vi "Boceto programa final.vi"() -> ()   [LabVIEW 2014]
panel:
  out "Gráfica":waveform(dbl)(graph)
  in  "Canal MATH":bool
  in  "VISA resource name":refnum<visa-resource-name>
  in  "Canal 1":bool
  in  "Canal 2":bool
  out "error out":errorcluster
  out "VISA resource name out":refnum<visa-resource-name>
  in  "error in (no error)":errorcluster
  out "Comando 4":string
  out "Medidas":string
  out "Comando 2":string
  out "Comando 1":string
  in  "Estilo de onda":u16(ring) items=["Puntos", "Vectores"]
  in  "Invertir colores":bool
  in  "Formato (YT o XY)":u16(ring) items=["YT", "XY"]
  in  "Contraste":i32(knob)=63 scale=0.0..100.0
  in  "Invertir canal":bool
  in  "Posición horizontal":i32(knob) scale=-5.0..5.0
  in  "Posición vertical":i32(knob) scale=-5.0..5.0
  in  "Escala vertical (V)":u16(ring) items=["2 mV", "5 mV", "10 mV", "20 mV", "50  mV", "100 mV", "200 mV", "500 mV", "1 V", "2 V", "5 V"]
  in  "Escala horizontal (s)":u16(ring) items=["25 n", "50 n", "100 n", "250 n", "500 n", "1 u", "2,5 u", "5 u", "10 u", "25 u", "50 u", "100 u", "250 u", "500 u", "1 m", "2,5 m", "5 m", "10 m", "25 m", "50 m", "100 m", "250 m", "500 m", "1 ", "2,5", "5", "10", "25", "50"]
  in  "Operaciones \ncon las señales":u16(ring)=1 items=["CH1 + CH2"=1, "CH1 - CH2"=2, "CH2 - CH1"=3, "CH1 * CH2"=4]
  in  "Acomplamiento":u16(ring) items=["AC", "DC", "GROUND"]
  in  "Selección de canal":u16(ring) items=["Canal 1", "Canal 2"]
  in  "Atenuación":u16(ring) items=["x1", "x10", "x20", "x50", "x100", "x500", "x1000"]
  in  "Ancho de banda":u16(ring)=1 items=["ON", "OFF"]
  out "Selección canal":string
  out "Comando concatenado":string
  in  "stop":bool
  out "Comando final":string
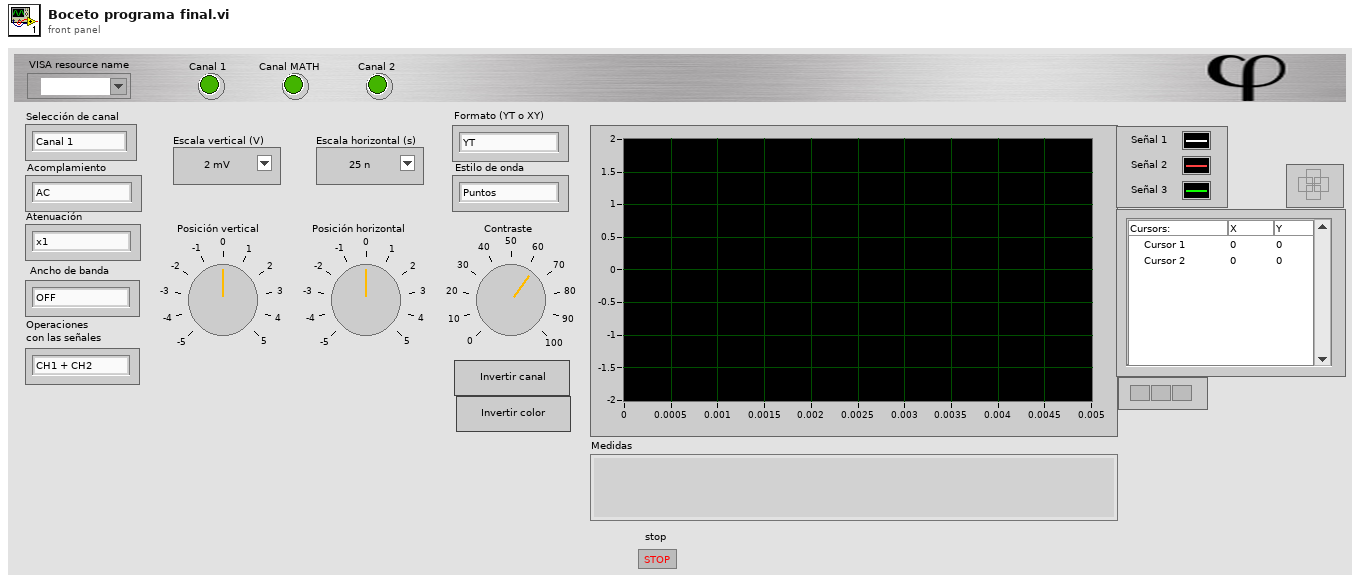
[diagram p1: front panel]
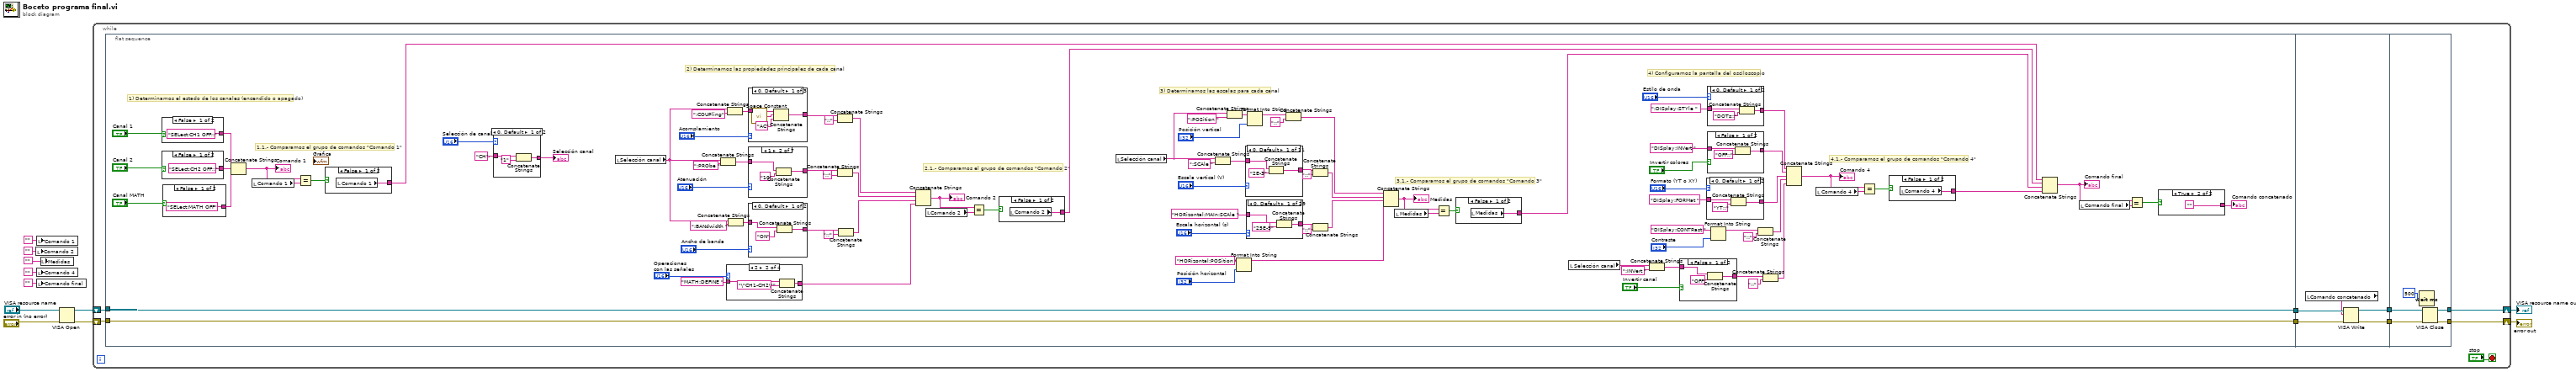
[diagram p0: block diagram]
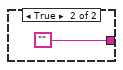
[diagram p2: hidden frame]
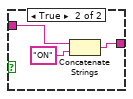
[diagram p3: hidden frame]
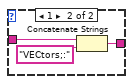
[diagram p4: hidden frame]
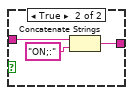
[diagram p5: hidden frame]
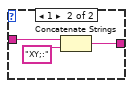
[diagram p6: hidden frame]
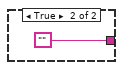
[diagram p7: hidden frame]
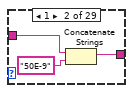
[diagram p8: hidden frame]
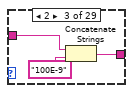
[diagram p9: hidden frame]
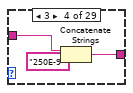
[diagram p10: hidden frame]
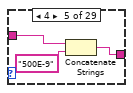
[diagram p11: hidden frame]
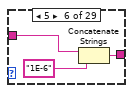
[diagram p12: hidden frame]
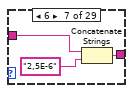
[diagram p13: hidden frame]
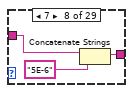
[diagram p14: hidden frame]
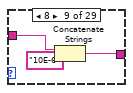
[diagram p15: hidden frame]
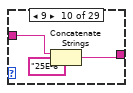
[diagram p16: hidden frame]
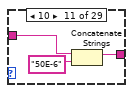
[diagram p17: hidden frame]
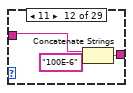
[diagram p18: hidden frame]
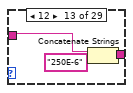
[diagram p19: hidden frame]
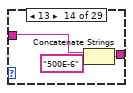
[diagram p20: hidden frame]
diagram:
  n1 = local write "Comando 2"("") -> ()
  n2 = local write "Comando 1"("") -> ()
  n3 = local write "Comando 4"("") -> ()
  n4 = local write "Comando final"("") -> ()
  n5 = local write "Medidas"("") -> ()
  n6 = VISA Open(error in (no error)="error in (no error)", VISA resource name="VISA resource name") -> (VISA resource name=w11:refnum<visa-resource-name>, error out=w10:errorcluster)  [unwired: 3 in]
  n7 = while {
    shift-right: [w13] -> w9
    shift-left: w11 -> [w18]
    shift-right: [w12] -> w8
    shift-left: w10 -> [w17]
    stop <- "stop" stop-if-true
    n8 = flat-sequence {
      tunnel: w18 -> [w114]
      tunnel: w17 -> [w113]
      tunnel: [w114] -> w20
      tunnel: [w113] -> w19
      tunnel: [w333] -> w15
      tunnel: w19 -> [w336]
      tunnel: w20 -> [w337]
      tunnel: [w334] -> w14
      tunnel: w15 -> [w338]
      tunnel: w14 -> [w339]
      tunnel: [w339] -> w13
      tunnel: [w338] -> w12
      frame #0 {
        # "1) Determinamos el estado de los canales (encendido o apagado)"
        # "4.1.- Comparamos el grupo de comandos \"Comando 4\""
        # "4) Configuramos la pantalla del osciloscopio"
        # "3.1.- Comparamos el grupo de comandos \"Comando 3\""
        # "3) Determinamos las escalas para cada canal"
        # "2.1.- Comparamos el grupo de comandos \"Comando 2\""
        # "1.1.- Comparamos el grupo de comandos \"Comando 1\""
        # "2) Determinamos las propiedades principales de cada canal"
        n9 = case shown="False" "Canal 1" {
          tunnel: ["SELect:CH1 OFF;:" "SELect:CH1 ON;:"] -> w107
          frame False {
          }
          frame True {
          }
        }
        n10 = case shown="False" "Canal 2" {
          tunnel: ["SELect:CH2 OFF;:" "SELect:CH2 ON;:"] -> w106
          frame False {
          }
          frame True {
          }
        }
        n11 = case shown="False" "Canal MATH" {
          tunnel: ["SELect:MATH OFF" "SELect:MATH ON"] -> w105
          frame False {
          }
          frame True {
          }
        }
        n12 = Concatenate Strings(w107, w106, w105) -> (w104:string)
        "Comando 1" <- w104
        n13 = local read "Comando 1"() -> (w103:string)
        n14 = Equal?(x=w104, y=w103) -> (x = y?=w102:bool)
        n15 = case shown="False" w102 {
          tunnel: [w317 ""] -> w33
          frame False {
            n16 = local read "Comando 1"() -> (w317:string)
          }
          frame True {
          }
        }
        n17 = case shown="0, Default" "Selección de canal" {
          tunnel: "CH" -> [w327 w330]
          tunnel: [w325 w328] -> w109
          frame 0, Default {
            n18 = Concatenate Strings(w327, "1") -> (w325:string)
          }
          frame 1 {
            n19 = Concatenate Strings(w330, "2") -> (w328:string)
          }
        }
        "Selección canal" <- w109
        n20 = local read "Selección canal"() -> (w84:string)
        n21 = Concatenate Strings(w84, ":PRObe ") -> (w98:string)
        n22 = case shown="2" "Operaciones \ncon las señales" {
          tunnel: "MATH:DEFINE " -> [w268 w271 w273 w276]
          tunnel: [w266 w270 w272 w275] -> w29
          frame 1, Default {
            n23 = Concatenate Strings(w268, "\"CH1+CH2\"") -> (w266:string)
          }
          frame 2 {
            n24 = Concatenate Strings(w271, "\"CH1-CH2\"") -> (w270:string)
          }
          frame 3 {
            n25 = Concatenate Strings(w273, "\"CH2-CH1\"") -> (w272:string)
          }
          frame 4 {
            n26 = Concatenate Strings(w276, "\"CH1*CH2\"") -> (w275:string)
          }
        }
        n27 = Concatenate Strings(w84, ":COUPling") -> (w101:string)
        n28 = Concatenate Strings(w84, ":BANdwidth ") -> (w96:string)
        n29 = case shown="1" "Atenuación" {
          tunnel: w98 -> [w285 w289 w291 w294 w297 w300 w303]
          tunnel: [w284 w287 w290 w293 w296 w299 w302] -> w87
          frame 0, Default {
            n30 = Concatenate Strings(w285, "1") -> (w284:string)
          }
          frame 1 {
            n31 = Concatenate Strings(w289, "10") -> (w287:string)
          }
          frame 2 {
            n32 = Concatenate Strings(w291, "20") -> (w290:string)
          }
          frame 3 {
            n33 = Concatenate Strings(w294, "50") -> (w293:string)
          }
          frame 4 {
            n34 = Concatenate Strings(w297, "100") -> (w296:string)
          }
          frame 5 {
            n35 = Concatenate Strings(w300, "500") -> (w299:string)
          }
          frame 6 {
            n36 = Concatenate Strings(w303, "1000") -> (w302:string)
          }
        }
        n37 = case shown="0, Default" "Ancho de banda" {
          tunnel: w96 -> [w280 w283]
          tunnel: [w278 w281] -> w85
          frame 0, Default {
            n38 = Concatenate Strings(w280, "ON") -> (w278:string)
          }
          frame 1 {
            n39 = Concatenate Strings(w283, "OFF") -> (w281:string)
          }
        }
        n40 = case shown="0, Default" "Acomplamiento" {
          tunnel: w101 -> [w306 w309 w314]
          tunnel: [w305 w310 w313] -> w90
          frame 0, Default {
            n41 = call <vilib>:"Space Constant.vi"() -> ("String"=w307:string)
            n42 = Concatenate Strings(w306, w307, "AC") -> (w305:string)
          }
          frame 1 {
            n43 = call <vilib>:"Space Constant.vi"() -> ("String"=w311:string)
            n44 = Concatenate Strings(w309, w311, "DC") -> (w310:string)
          }
          frame 2 {
            n45 = call <vilib>:"Space Constant.vi"() -> ("String"=w315:string)
            n46 = Concatenate Strings(w314, w315, "GND") -> (w313:string)
          }
        }
        n47 = Concatenate Strings(w90, ";:") -> (w28:string)
        n48 = Concatenate Strings(w87, ";:") -> (w27:string)
        n49 = Concatenate Strings(w85, ";:") -> (w26:string)
        n50 = Concatenate Strings(w28, w27, w26, w29) -> (w81:string)
        "Comando 2" <- w81
        n51 = local read "Comando 2"() -> (w82:string)
        n52 = Equal?(x=w81, y=w82) -> (x = y?=w83:bool)
        n53 = case shown="False" w83 {
          tunnel: [w264 ""] -> w32
          frame False {
            n54 = local read "Comando 2"() -> (w264:string)
          }
          frame True {
          }
        }
        n55 = local read "Selección canal"() -> (w67:string)
        n56 = Concatenate Strings(w67, ":SCAle ") -> (w71:string)
        n57 = Concatenate Strings(w67, ":POSition ") -> (w68:string)
        n58 = Format Into String(initial string="HORizontal:POSition ", "Posición horizontal") -> (resulting string=w76:string)  [unwired: 2 in, 1 out]
        n59 = case shown="0, Default" "Escala vertical (V)" {
          tunnel: w71 -> [w232 w236 w238 w241 w244 w247 w249 w253 w256 w259 w262]
          tunnel: [w231 w234 w237 w240 w243 w246 w250 w252 w255 w258 w261] -> w63
          frame 0, Default {
            n60 = Concatenate Strings(w232, "2E-3") -> (w231:string)
          }
          frame 1 {
            n61 = Concatenate Strings(w236, "5E-3") -> (w234:string)
          }
          frame 2 {
            n62 = Concatenate Strings(w238, "10E-3 ") -> (w237:string)
          }
          frame 3 {
            n63 = Concatenate Strings(w241, "20E-3") -> (w240:string)
          }
          frame 4 {
            n64 = Concatenate Strings(w244, "50E-3") -> (w243:string)
          }
          frame 5 {
            n65 = Concatenate Strings(w247, "100E-3") -> (w246:string)
          }
          frame 6 {
            n66 = Concatenate Strings(w249, "200E-3") -> (w250:string)
          }
          frame 7 {
            n67 = Concatenate Strings(w253, "500E-3") -> (w252:string)
          }
          frame 8 {
            n68 = Concatenate Strings(w256, "1") -> (w255:string)
          }
          frame 9 {
            n69 = Concatenate Strings(w259, "2") -> (w258:string)
          }
          frame 10 {
            n70 = Concatenate Strings(w262, "5") -> (w261:string)
          }
        }
        n71 = case shown="0, Default" "Escala horizontal (s)" {
          tunnel: "HORizontal:MAIn:SCAle " -> [w145 w149 w151 w154 w157 w160 w163 w166 w169 w172 w175 w177 w180 w183 w186 w189 w192 w195 w198 w201 w204 w207 w210 w213 w216 w219 w222 w225 w228]
          tunnel: [w144 w147 w150 w153 w156 w159 w164 w165 w168 w171 w174 w178 w181 w184 w187 w190 w193 w196 w199 w202 w205 w208 w211 w214 w217 w220 w223 w226 w229] -> w65
          frame 0, Default {
            n72 = Concatenate Strings(w145, "25E-9") -> (w144:string)
          }
          frame 1 {
            n73 = Concatenate Strings(w149, "50E-9") -> (w147:string)
          }
          frame 2 {
            n74 = Concatenate Strings(w151, "100E-9") -> (w150:string)
          }
          frame 3 {
            n75 = Concatenate Strings(w154, "250E-9") -> (w153:string)
          }
          frame 4 {
            n76 = Concatenate Strings(w157, "500E-9") -> (w156:string)
          }
          frame 5 {
            n77 = Concatenate Strings(w160, "1E-6") -> (w159:string)
          }
          frame 6 {
            n78 = Concatenate Strings(w163, "2,5E-6") -> (w164:string)
          }
          frame 7 {
            n79 = Concatenate Strings(w166, "5E-6") -> (w165:string)
          }
          frame 8 {
            n80 = Concatenate Strings(w169, "10E-6") -> (w168:string)
          }
          frame 9 {
            n81 = Concatenate Strings(w172, "25E-6") -> (w171:string)
          }
          frame 10 {
            n82 = Concatenate Strings(w175, "50E-6") -> (w174:string)
          }
          frame 11 {
            n83 = Concatenate Strings(w177, "100E-6") -> (w178:string)
          }
          frame 12 {
            n84 = Concatenate Strings(w180, "250E-6") -> (w181:string)
          }
          frame 13 {
            n85 = Concatenate Strings(w183, "500E-6") -> (w184:string)
          }
          frame 14 {
            n86 = Concatenate Strings(w186, "1E-3") -> (w187:string)
          }
          frame 15 {
            n87 = Concatenate Strings(w189, "2,5E-3") -> (w190:string)
          }
          frame 16 {
            n88 = Concatenate Strings(w192, "5E-3") -> (w193:string)
          }
          frame 17 {
            n89 = Concatenate Strings(w195, "10E-3") -> (w196:string)
          }
          frame 18 {
            n90 = Concatenate Strings(w198, "25E-3") -> (w199:string)
          }
          frame 19 {
            n91 = Concatenate Strings(w201, "50E-3") -> (w202:string)
          }
          frame 20 {
            n92 = Concatenate Strings(w204, "100E-3") -> (w205:string)
          }
          frame 21 {
            n93 = Concatenate Strings(w207, "250E-3") -> (w208:string)
          }
          frame 22 {
            n94 = Concatenate Strings(w210, "500E-3") -> (w211:string)
          }
          frame 23 {
            n95 = Concatenate Strings(w213, "1E0") -> (w214:string)
          }
          frame 24 {
            n96 = Concatenate Strings(w216, "2,5E0") -> (w217:string)
          }
          frame 25 {
            n97 = Concatenate Strings(w219, "5E0") -> (w220:string)
          }
          frame 26 {
            n98 = Concatenate Strings(w222, "10E0") -> (w223:string)
          }
          frame 27 {
            n99 = Concatenate Strings(w225, "25E0") -> (w226:string)
          }
          frame 28 {
            n100 = Concatenate Strings(w228, "50E0") -> (w229:string)
          }
        }
        n101 = Format Into String(initial string=w68, "Posición vertical") -> (resulting string=w74:string)  [unwired: 2 in, 1 out]
        n102 = Concatenate Strings(w74, ";:") -> (w24:string)
        n103 = Concatenate Strings(w63, ";:") -> (w25:string)
        n104 = Concatenate Strings(w65, ";:") -> (w64:string)
        n105 = Concatenate Strings(w24, w25, w64, w76) -> (w59:string)
        "Medidas" <- w59
        n106 = local read "Medidas"() -> (w61:string)
        n107 = Equal?(x=w59, y=w61) -> (x = y?=w60:bool)
        n108 = case shown="False" w60 {
          tunnel: [w142 ""] -> w31
          frame False {
            n109 = local read "Medidas"() -> (w142:string)
          }
          frame True {
          }
        }
        n110 = local read "Selección canal"() -> (w41:string)
        n111 = Concatenate Strings(w41, ":INVert ") -> (w46:string)
        n112 = case shown="False" "Invertir canal" {
          tunnel: w46 -> [w119 w122]
          tunnel: [w118 w121] -> w43
          frame False {
            n113 = Concatenate Strings(w119, "OFF") -> (w118:string)
          }
          frame True {
            n114 = Concatenate Strings(w122, "ON") -> (w121:string)
          }
        }
        n115 = case shown="0, Default" "Formato (YT o XY)" {
          tunnel: "DISplay:FORMat " -> [w138 w140]
          tunnel: [w136 w139] -> w48
          frame 0, Default {
            n116 = Concatenate Strings(w138, "YT;:") -> (w136:string)
          }
          frame 1 {
            n117 = Concatenate Strings(w140, "XY;:") -> (w139:string)
          }
        }
        n118 = case shown="0, Default" "Estilo de onda" {
          tunnel: ":DISplay:STYle " -> [w126 w128]
          tunnel: [w124 w127] -> w50
          frame 0, Default {
            n119 = Concatenate Strings(w126, "DOTs;:") -> (w124:string)
          }
          frame 1 {
            n120 = Concatenate Strings(w128, "VECtors;:") -> (w127:string)
          }
        }
        n121 = case shown="False" "Invertir colores" {
          tunnel: "DISplay:INVert " -> [w131 w134]
          tunnel: [w130 w133] -> w49
          frame False {
            n122 = Concatenate Strings(w131, "OFF;:") -> (w130:string)
          }
          frame True {
            n123 = Concatenate Strings(w134, "ON;:") -> (w133:string)
          }
        }
        n124 = Format Into String(initial string="DISplay:CONTRast ", "Contraste") -> (resulting string=w39:string)  [unwired: 2 in, 1 out]
        n125 = Concatenate Strings(w39, ";:") -> (w38:string)
        n126 = Concatenate Strings(w43, ";:") -> (w42:string)
        n127 = Concatenate Strings(w50, w49, w48, w38, w42) -> (w35:string)
        "Comando 4" <- w35
        n128 = local read "Comando 4"() -> (w36:string)
        n129 = Equal?(x=w35, y=w36) -> (x = y?=w37:bool)
        n130 = case shown="False" w37 {
          tunnel: [w116 ""] -> w34
          frame False {
            n131 = local read "Comando 4"() -> (w116:string)
          }
          frame True {
          }
        }
        n132 = Concatenate Strings(w33, w32, w31, w34) -> (w30:string)
        "Comando final" <- w30
        n133 = local read "Comando final"() -> (w112:string)
        n134 = Equal?(x=w30, y=w112) -> (x = y?=w115:bool)
        n135 = case shown="True" w115 {
          tunnel: [w331 ""] -> w111
          frame False {
            n136 = local read "Comando final"() -> (w331:string)
          }
          frame True {
          }
        }
        "Comando concatenado" <- w111
      }
      frame #1 {
        n137 = local read "Comando concatenado"() -> (w335:string)
        n138 = VISA Write(VISA resource name=w337, write buffer=w335, error in (no error)=w336) -> (VISA resource name out=w334:refnum<visa-resource-name>, error out=w333:errorcluster)  [unwired: 1 out]
      }
      frame #2 {
        n139 = Wait (ms)(milliseconds to wait=u32 500 ("millisecond multiple")) -> ()  [unwired: 1 out]
      }
    }
  }
  "VISA resource name out" <- w9
  "error out" <- w8
  n140 = VISA Close(VISA resource name=w9, error in (no error)=w8) -> ()  [unwired: 1 out]
